vi "Termostato.vi"() -> ()   [LabVIEW 2020]
panel:
  in  "stop":bool
  out "Caldaia":bool
  out "Temp":dbl
  out "Waveform Chart":dynamicdata(graph)
  in  "Tensione":dbl(slide) scale=0.0..3.0
  in  "SV":dbl
  in  "IST":dbl
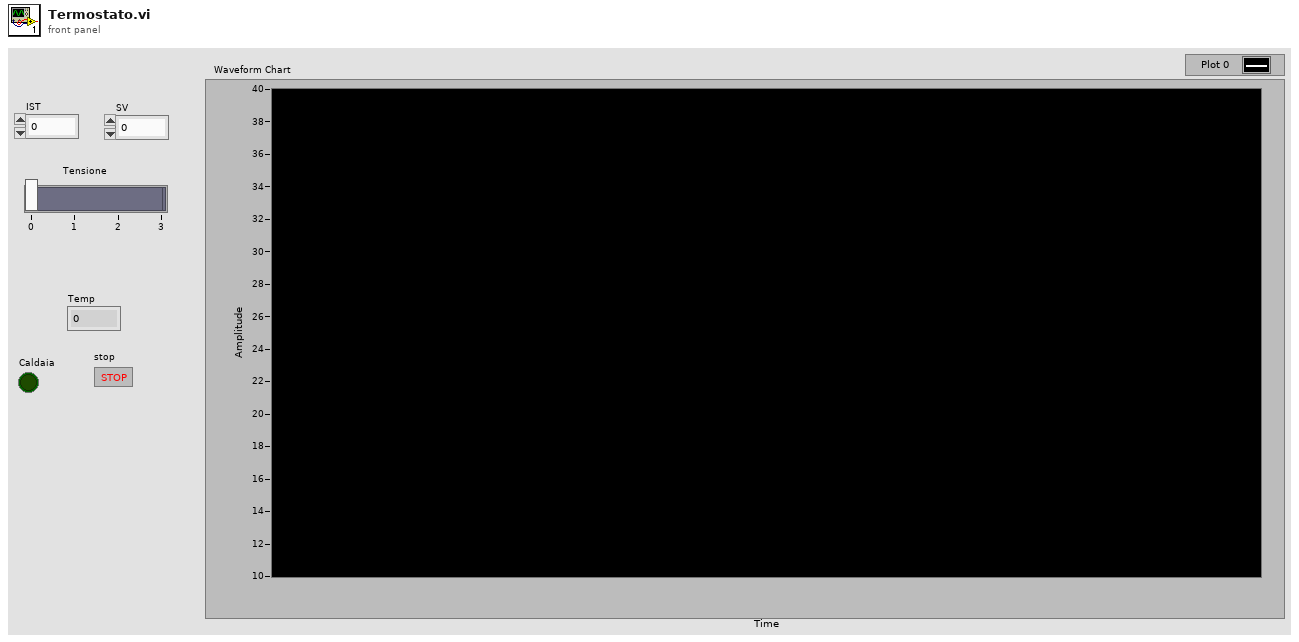
[diagram p1: front panel]
types:
  T1 = typedef "imagedata.ctl" = cluster{"image type":i32, "image depth":i32, "image":u8[], "mask":u8[], "colors":u32[], "Rectangle":cluster{"left":i16, "top":i16, "right":i16, "bottom":i16}}
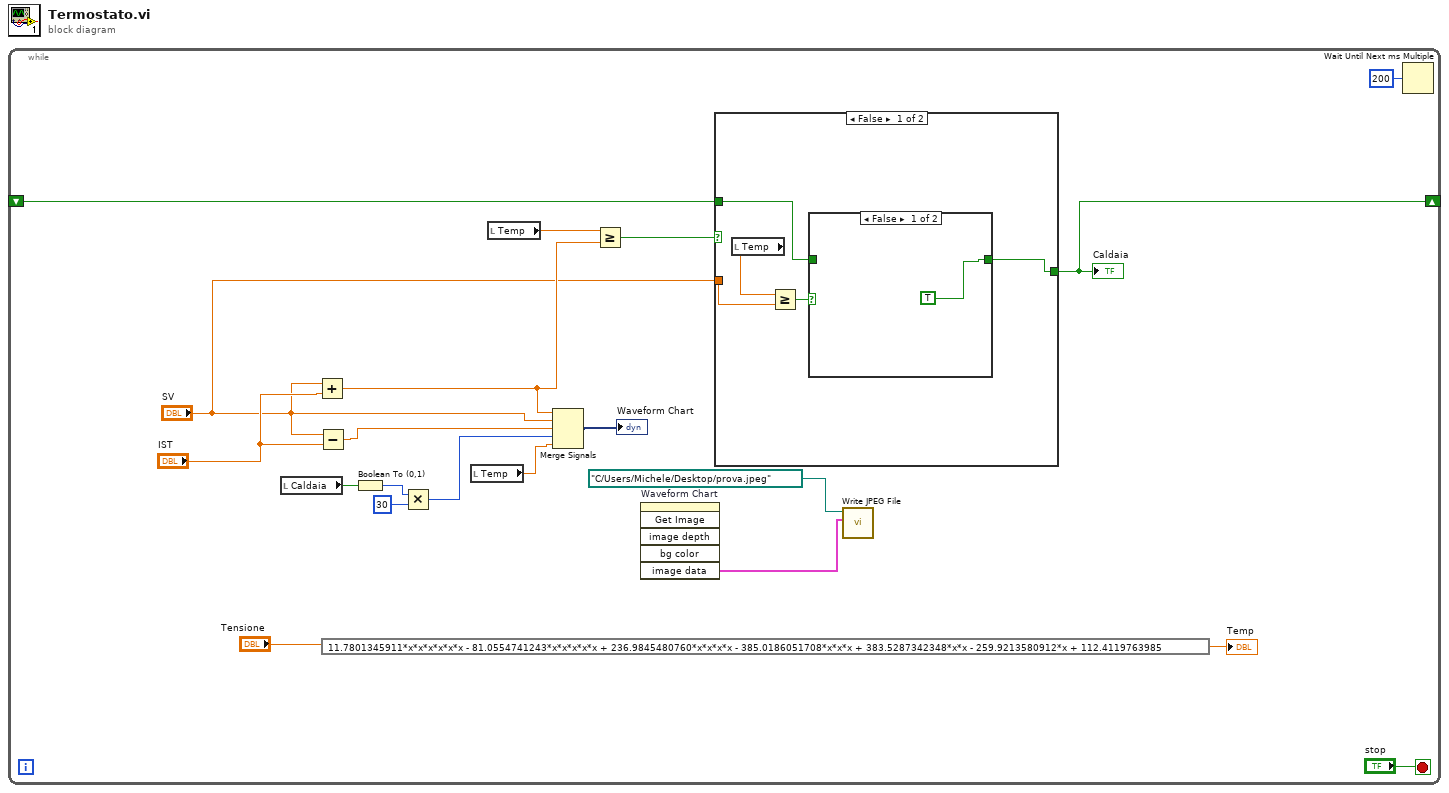
[diagram p0: block diagram]
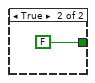
[diagram p3: hidden frame]
diagram:
  n1 = while {
    shift-right: [w6] -> _
    shift-left: _ -> [w5]
    stop <- "stop" stop-if-true
    n2 = local read "Caldaia"() -> (w15:bool)
    n3 = Add(x="SV", y="IST") -> (x+y=w10:dbl)
    n4 = Subtract(x="SV", y="IST") -> (x-y=w16:dbl)
    n5 = expression code="11.7801345911*x*x*x*x*x*x - 81.0554741243*x*x*x*x*x + 236.9845480760*x*x*x*x - 385.0186051708*x*x*x + 383.5287342348*x*x - 259.9213580912*x + 112.4119763985"("Tensione") -> (→"Temp":dbl)
    n6 = Boolean To (0,1)(Boolean=w15) -> (0, 1=w14:i16)
    n7 = Multiply(x=w14, y=i16 30) -> (x*y=w12:i16)
    n8 = local read "Temp"() -> (w11:dbl)
    n9 = local read "Temp"() -> (w8:dbl)
    n10 = Merge Signals(w10, "SV", w16, w12, w11) -> (→"Waveform Chart":dynamicdata)
    n11 = Greater Or Equal?(x=w8, y=w10) -> (x >= y?=w9:bool)
    n12 = invoke on="Waveform Chart" class="WFChart (strict)" method="Get Image"() -> ("image data"=w1:T1)  [unwired: 6 in, 5 out]
    n13 = case shown="False" w9 {
      tunnel: [w22 FALSE] -> w6
      tunnel: "SV" -> [w24 _]
      tunnel: w5 -> [w21 _]
      frame False {
        n14 = local read "Temp"() -> (w25:dbl)
        n15 = Greater Or Equal?(x=w25, y=w24) -> (x >= y?=w23:bool)
        n16 = case shown="False" w23 {
          tunnel: [TRUE w27] -> w22
          tunnel: w21 -> [_ w27]
          frame False {
          }
          frame True {
          }
        }
      }
      frame True {
      }
    }
    "Caldaia" <- w6
    n17 = call <vilib>:"Write JPEG File.vi"("image data"=w1, "path to JPEG file"=path "C:/Users/Michele/Desktop/prova.jpeg") -> ()  [unwired: 8 in, 2 out]
    n18 = Wait Until Next ms Multiple(millisecond multiple=u32 200) -> ()  [unwired: 1 out]
  }
